vi "GUI_TestStand.vi"() -> ()   [LabVIEW 2011]
uses:
  <vilib>/vision/Image Controls.llb/IMAQ Image.ctl
panel:
  in  "delay.Channel_D::8":dbl=40.15 caption="Discharge delay D" format="%_4f"
  in  "delay.Channel_C::8":dbl=40.15 caption="Discharge delay C" format="%_4f"
  in  "delay.Channel_B::8":dbl=40.15 caption="Discharge delay B" format="%_4f"
  in  "GUIdevice 8":string="TS-dg535-2"
  in  "delay.Channel_A::8":dbl=40.15 caption="Discharge delay A" format="%_4f"
  in  "delay.Channel_D::5":dbl=40.15 caption="Discharge delay D" format="%_4f"
  in  "delay.Channel_C::5":dbl=40.15 caption="Discharge delay C" format="%_4f"
  in  "delay.Channel_B::5":dbl=40.15 caption="Discharge delay B" format="%_4f"
  in  "GUIdevice 5":string="TS-dg535-1"
  in  "delay.Channel_A::5":dbl=40.15 caption="Discharge delay A" format="%_4f"
  in  "localsavingpath::2":path
  in  "save::2":bool
  in  "gain::2":dbl=0.001 caption="Gain" format="%_4f"
  in  "triggerdelay::2":dbl=0.001 caption="Trigger delay" format="%_4f"
  out "image::2":T1(plugin-control) caption="Mode1"
  in  "centroidy::2":dbl=0.001 caption="centroid y" format="%_4f"
  in  "centroidx::2":dbl=0.001 caption="centroid x" format="%_4f"
  in  "exposure::2":dbl=0.001 caption="exposure" format="%_4f"
  in  "GUIdevice 2":string="TS-Mode1"
  in  "highspeed::4":dbl=25.5 caption="Arcus 2 Hispeed" format="%_4f"
  in  "highspeed::3":dbl=25.5 caption="Arcus 1 Hispeed" format="%_4f"
  in  "wangle::1":dbl caption="w" format="%_4f"
  in  "vangle::1":dbl caption="v" format="%_4f"
  in  "uangle::1":dbl=0.5 caption="u" format="%_4f"
  in  "Mode::7":bool
  in  "GUIdevice 7":string="TS-shotcontrol"
  in  "GUIdevice 6":string="TS-digitizer-1"
  in  "Test Cluster":T2 {"verticalrange::6" format="%_4f"}
  in  "ypos::1":dbl caption="y" format="%_4f"
  in  "GUIdevice 4":string="TSArcus2"
  in  "position::4":dbl=40.15 caption="Arcus 2 position" format="%_4f"
  in  "position::3":dbl=25.5 caption="Arcus 1 position" format="%_4f"
  in  "GUIdevice 3":string="TSArcus1"
  in  "zpos::1":dbl caption="z" format="%_4f"
  in  "GUIdevice 1":string="TS-hexapod"
  in  "insert tag":bool=TRUE
  in  "stop":bool
  in  "xpos::1":dbl=0.5 caption="x" format="%_4f"
  # "TEST STAND GRAPHICAL USER INTERFACE"
  # "StagingPXIFast1"
  # "TS-digitizer-1"
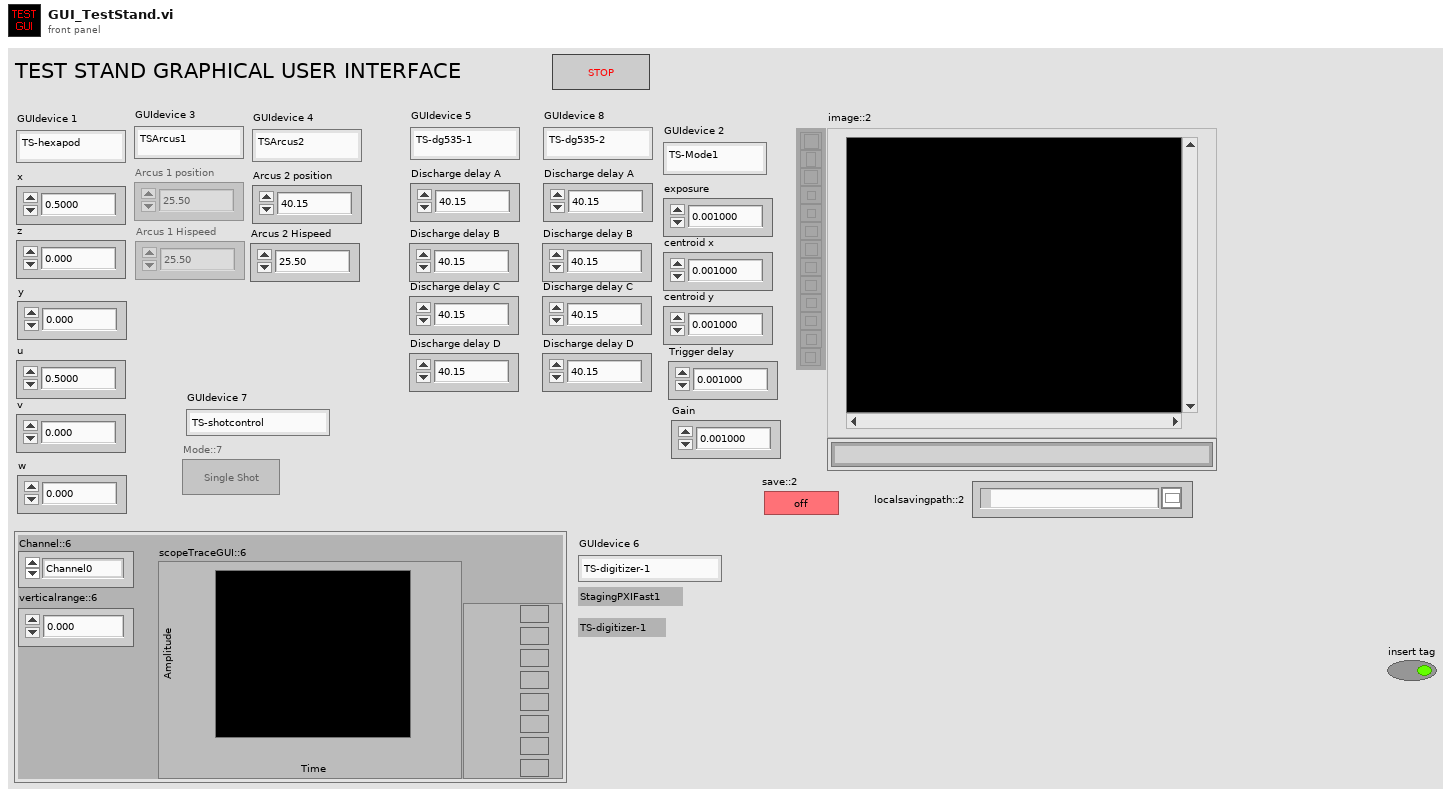
[diagram p1: front panel]
types:
  T1 = typedef "IMAQ Image.ctl" = refnum<image>
  T2 = cluster{"verticalrange::6":dbl, "Channel::6":enum16{"Channel0", "Channel1"}, "scopeTraceGUI::6":waveform(dbl)[]}
  T3 = typedef "EventTypDef.ctl" = refnum<user-event>
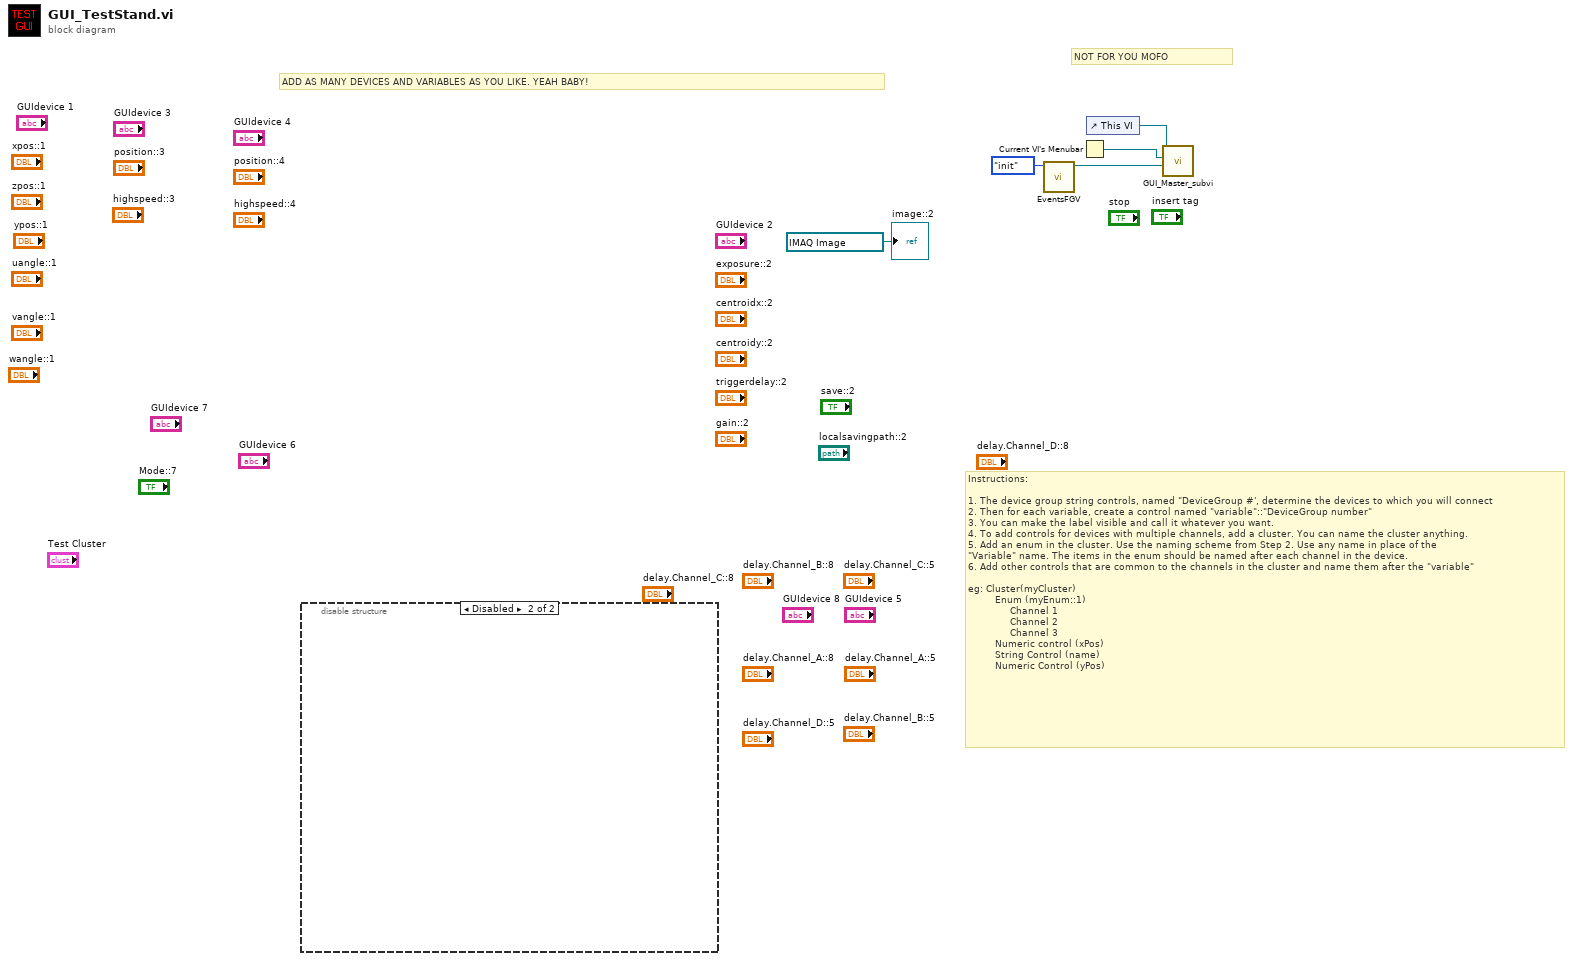
[diagram p0: block diagram]
diagram:
  # "Instructions:\n\n1. The device group string controls, named \"DeviceGroup #', determine the devices to which you will connect\n2. Then for each variable, create a control named \"variable\"::\"DeviceGroup number\"\n3. You can make the label visible and call it whatever you want.\n4. To add controls for devices with multiple channels, add a cluster. You can name the cluster anything.\n5. Add an enum in the cluster. Use the naming scheme from Step 2. Use any name in place of the \n\"Variable\" name. The items in the enum should be named after each channel in the device. \n6. Add other controls that are common to the channels in the cluster and name them after the \"variable\"\n\neg: Cluster(myCluster)\n         Enum (myEnum::1)\n              Channel 1 \n              Channel 2\n              Channel 3\n         Numeric control (xPos)\n         String Control (name)\n         Numeric Control (yPos)"
  # "ADD AS MANY DEVICES AND VARIABLES AS YOU LIKE. YEAH BABY!"
  # "NOT FOR YOU MOFO"
  n1 = disable-structure shown="Disabled" {
    frame Enabled {
    }
    frame Disabled {
    }
  }
  n2 = call "EventsFGV.vi"("Command"=enum16{"get", "init"}."init") -> ("New Event"=w2:T3)  [unwired: 9 in, 1 out]
  n3 = Current VI's Menubar() -> (w4:refnum<k9>)
  n4 = control-ref of="This VI"() -> (w5:refnum<vi>)
  n5 = call "GUI_Master_subvi.vi"("User Event"=w2, "Caller menu reference"=w4, "Caller VI ref"=w5) -> ()  [unwired: 9 in]
  "image::2" <- T1 refnum ("New Image")
